vi "Coherent cmnd pre-proc L1 (direct).vi"(10 "Coherent Commands":T2, 11 "Coherent laser commands L1":T1) -> (3 "concatenated string":string)   [LabVIEW 2020]
uses:
  Type defs/Coherent commands direct mode.ctl
  Type defs/Commands List.ctl
  Type defs/Coherent comms control.ctl
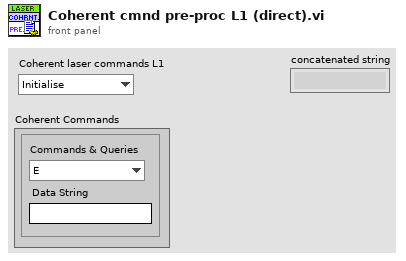
[diagram p1: front panel]
types:
  T1 = typedef "Coherent comms control.ctl" = enum16{"Initialise", "Get Command", "Set Command", "Clear Buffer", "Close"}
  T2 = typedef "Coherent commands direct mode.ctl" = cluster{"Commands & Queries":T3, "Data String":string}
  T3 = typedef "Commands List.ctl" = enum16{"E", "B", "FL", "HM", "L", "LBOH", "LBOOPT", "LFP", "PROMPT", "SM", "S", "VW", "VWS", "HB", "HBR", "REQ", "ALIGN", "K", "F", "FH", "UF", "PHLDC", "PZTMC", "PZTXC", "PZTYC", "PHLDP", "PZTMP", "PZTXP", "PZTYP", "PTRK", "MDLK", "PP", "TS", "STPRPOS", "C", "D1C", "D2C", "BT", "D1T", "D2T", "VT", "LBOT", "ET", "D1ST", "D2ST", "VST", "LBOST", "EST", "D1TD", "D2TD", "VD", "LBOD", "ED", "D1HST", "D2HST", "LRS", "D1SS", "D2SS", "VSS", "LBOSS", "ESS", "D1H", "D2H", "HH", "D1V", "D2V", "SV", "MB", "PI", "BV", "AMDLK", "PZTS", "TMAX", "TMIN", "ALIGNP", "ALIGNW", "PZTXCM", "PZTXCP", "PZTXPM", "PZTXPP", "PZTYCM", "PZTYCP", "PZTYPM", "PZTYPP", "RH", "SN", "ST", "GDDCURVE", "GDD", "GDDCURVEN", "SETCURVEN", "SETCURVEPT", "SAVECURVE", "DELCURVE", "CURVEN", "CURVEPT", "CURVE", "COMP", "HMCOMP", "GDDMAX", "GDDMIN"}
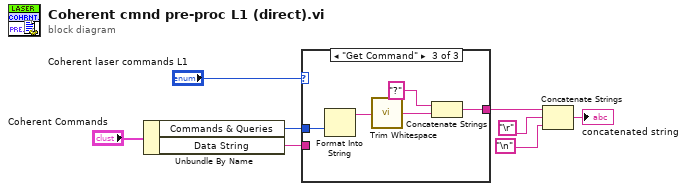
[diagram p0: block diagram]
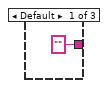
[diagram p2: hidden frame]
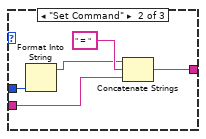
[diagram p3: hidden frame]
diagram:
  n1 = Unbundle By Name("Coherent Commands") -> ("Commands & Queries"=w7:T3, "Data String"=w1:string)
  n2 = case shown="\"Get Command\"" "Coherent laser commands L1" {
    tunnel: w7 -> [_ w11 w19]
    tunnel: ["" w13 w15] -> w3
    tunnel: w1 -> [_ w12 _]
    frame Default {
    }
    frame "Set Command" {
      n3 = Format Into String(w11) -> (resulting string=w10:string)  [unwired: 3 in, 1 out]
      n4 = Concatenate Strings(w10, " = " ("string"), w12) -> (w13:string)
    }
    frame "Get Command" {
      n5 = Format Into String(w19) -> (resulting string=w16:string)  [unwired: 3 in, 1 out]
      n6 = call <vilib>:"Trim Whitespace.vi"("string"=w16) -> ("trimmed string"=w17:string)  [unwired: 1 in]
      n7 = Concatenate Strings("?", w17) -> (w15:string)
    }
  }
  n8 = Concatenate Strings(w3, "\r", "\n") -> (→"concatenated string":string)
